vi "AllThingsNotes.vi"(8 "Choice":string) -> (0 "Text":string, 3 "Array":string[](array[string]))   [LabVIEW 2022 SP3]
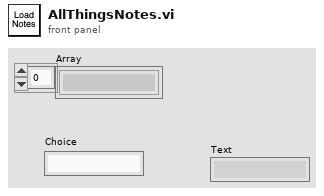
[diagram p1: front panel]
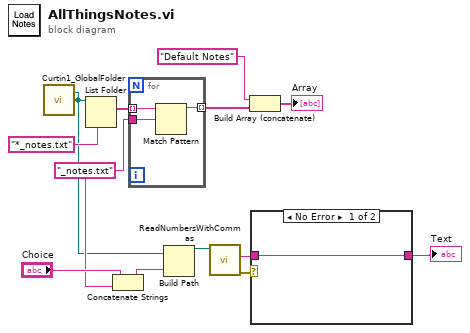
[diagram p0: block diagram]
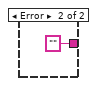
[diagram p2: hidden frame]
diagram:
  w7 = "_notes.txt" ("pattern")
  n1 = call "Curtin1_GlobalFolder.vi"() -> ("LabVIEW Data Path"=w4:path)  [unwired: 1 in, 1 out]
  n2 = List Folder(path=w4, pattern="*_notes.txt") -> (filenames=w12:string[])  [unwired: 2 in, 3 out]
  n3 = Concatenate Strings("Choice", w7) -> (w6:string)
  n4 = for {
    tunnel: w12 -> [w16] mode=indexing
    tunnel: w7 -> [w15]
    tunnel: [w14] -> w13 mode=indexing
    n5 = Match Pattern(string=w16, regular expression=w15) -> (before substring=w14:string)  [unwired: 1 in, 3 out]
  }
  n6 = Build Path(base path=w4, name or relative path=w6) -> (appended path=w1:path)
  n7 = call "ReadNumbersWithCommas.vi"("file (use dialog)"=w1) -> ("error out"=w3:errorcluster, "text"=w2:string)  [unwired: 7 in, 2 out]
  n8 = Build Array (concatenate)("Default Notes" ("string"), w13) -> (→"Array":string[])
  n9 = case shown="No Error" w3 {
    tunnel: [w17 ""] -> w5
    tunnel: w2 -> [w17 _]
    frame No Error {
    }
    frame Error {
    }
  }
  "Text" <- w5
